vi "Read Main UI.vi"(11 "Controller in":refnum<class "Controller.lvclass">) -> (2 "Main UI":refnum<class "Message Enqueuer.lvclass">, 3 "Controller out":refnum<class "Controller.lvclass">)   [LabVIEW 2011, in "Controller.lvclass"]
uses:
  Controller.lvclass
  <userlib>/_Frameworks/ActorFramework/Message Enqueuer/Message Enqueuer.lvclass
  Controller.lvclass/Controller.ctl
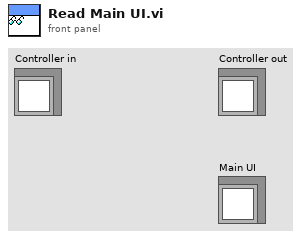
[diagram p1: front panel]
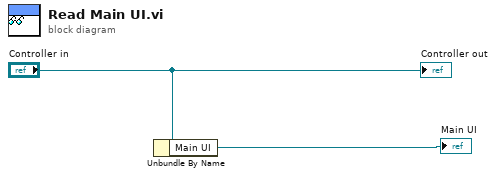
[diagram p0: block diagram]
diagram:
  n1 = Unbundle By Name("Controller in") -> ("Main UI"=→"Main UI":refnum<class "Message Enqueuer.lvclass">)
  "Controller out" <- "Controller in"
